vi "Save Known Packages.vi"(8 "error in (no error)":errorcluster, 11 "Package Array from File":T1[](array[typedef])) -> (0 "error out":errorcluster, 1 "Success?":bool)   [LabVIEW 2019]
doc: "Load package info from file."
uses:
  <vilib>/Utility/file.llb/Write Delimited Spreadsheet (string).vi
  Ctl/Ctl_Package Identifier Cluster.ctl
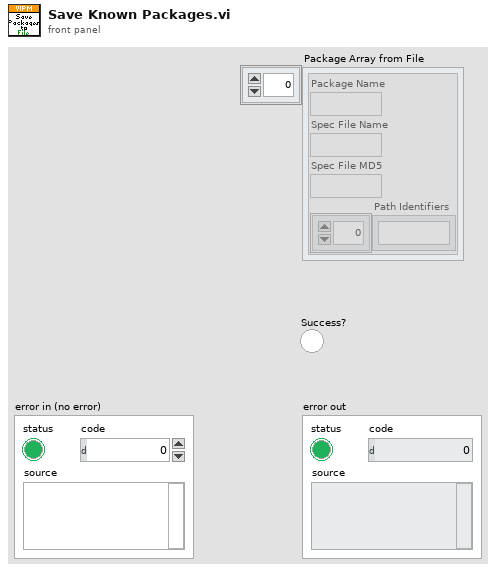
[diagram p1: front panel]
types:
  T1 = typedef "Ctl_Package Identifier Cluster.ctl" = cluster{"Package Name":string, "Spec File Name":string, "Spec File MD5":string, "Path Identifiers":string[]}
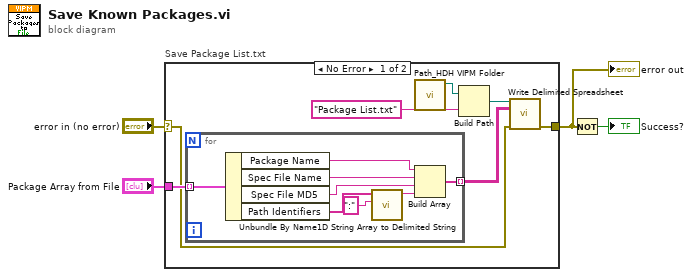
[diagram p0: block diagram]
diagram:
  n1 = case "Save Package List.txt" shown="No Error" "error in (no error)" {
    selector: "error in (no error)" -> [w9 w20]
    tunnel: "Package Array from File" -> [w11 _]
    tunnel: [w8 w20] -> w2
    frame No Error {
      n2 = for {
        tunnel: w11 -> [w19] mode=indexing
        tunnel: [w12] -> w10 mode=indexing
        n3 = Unbundle By Name(w19) -> ("Package Name"=w18:string, "Spec File Name"=w17:string, "Spec File MD5"=w16:string, "Path Identifiers"=w15:string[])
        n4 = call <vilib>:"1D String Array to Delimited String.vi"("delimiter"=":", "string array"=w15) -> ("delimited string"=w13:string)  [unwired: 9 in]
        n5 = Build Array(w18, w17, w16, w13) -> (w12:string[])
      }
      n6 = call "Path_HDH VIPM Folder.vi"() -> ("HDH\\VIPM path"=w7:path)  [unwired: 10 in, 1 out]
      n7 = Build Path(base path=w7, name or relative path="Package List.txt") -> (appended path=w5:path)
      n8 = call-poly <vilib>:"Write Delimited Spreadsheet.vi"("file path (dialog if empty)"=w5, "2D data"=w10, "error in (no error)"=w9) -> ("error out"=w8:errorcluster)  [unwired: 11 in, 1 out]
    }
    frame Error {
    }
  }
  "error out" <- w2
  n9 = Not(x=w2) -> (.not. x?=→"Success?":bool)
